vi "Main.vi"(11 "Module Admin":refnum<class "Delacor_lib_QMH_Module Admin.lvclass">) -> ()   [LabVIEW 2016, in "Impedance Data Acquisition and Decoding.lvlib"]
doc: "This template is based off of the Queued Message Handler design pattern and the Queued Message Handler project template that ships with LabVIEW.\n\nThe main difference is that the queue is private to this module and communication between modules is performed via Broadcast and Request events.\n\nRequest events are wrapped in public API methods and are handled in the Event Handling Loop (EHL) of this VI. Any module can register for Broadcast events sent by this module. The EHL generates messages based on user interface actions.\n\nThe Message Handling Loop (MHL) processes messages generated by the EHL, or by other messages. The messages are string values, so new messages can be added easily to the Message Cases case structure in the MHL. Each message cluster can also provide an optional value for Message Data, which is a variant that can be converted to whatever message-specific data is required.\n_____\nBased on Delacor QMH Project Template 5.0.0.82."
uses:
  Impedance Data Acquisition and Decoding.lvlib
  Module Data--cluster.ctl
  <vilib>/Delacor/Delacor QMH/Libraries/Message Queue_class/Delacor_lib_QMH_Message Queue.lvclass
  <vilib>/Delacor/Delacor QMH/Libraries/Message Queue_class/Delacor_lib_QMH_Enqueue Message (Single).vi
  <vilib>/ErrorRing/Error Ring.xnode
  <vilib>/Utility/error.llb/Error Cluster From Error Code.vi
  <vilib>/Delacor/Delacor QMH/Libraries/Module Admin_class/Delacor_lib_QMH_Module Admin.lvclass
  Stop Argument--cluster.ctl
  <vilib>/Utility/miscctls.llb/LVPointTypeDef.ctl
  Stop Acquiring Argument--cluster.ctl
  BusA/FINS3-E BusA Data Acquisition and Decoding/BusA Hardware Configuration.ctl
  FINS-3E Settings Editor/Settings--cluster.ctl
  FINS-3E Settings Editor/Update Application Settings (Reply Payload)--cluster.ctl
  BusB Typedef.ctl
  BusB Hardware Configuration.ctl
  Start Acquiring (Reply Payload)--cluster.ctl
  Start Acquiring Argument--cluster.ctl
  BusD/FINS3-E BusD Data Acquisition and Decoding/BusD Hardware Configuration.ctl
  FINS-3E Settings Editor/Logging Configuration.ctl
  BusB Initialization Parameters.ctl
  BusA/FINS3-E BusA Data Acquisition and Decoding/FCC Parameters.ctl
  IMU/FINS3-E IMU Data Acquisition and Decoding/FINS3-E IMU Hardware Configuration.ctl
  Configurator/FINS3-E Config Hardware Configuration.ctl
  AC 1553/FINS3-E AC Data Acquisition and Decoding/Aircraft Bus Hardware Configuration.ctl
  TERCOM/FINS3-E TERCOM Data Acquisition and Decoding/TERCOM Hardware Configuration.ctl
  DSMAC/FINS3-E DSMAC Data Acquisition and Decoding/DSMAC Hardware Configuration.ctl
  FINS3-E TEL Bus/GPS Hardware Configuration.ctl
  Initialize FINS for FTR Argument--cluster.ctl
  Initialize FINS for Qualification Argument--cluster.ctl
  Settings Editor/Settings Editor.lvlib
  Acquisition/Reg_Map.ctl
  Acquisition/Acquisition.lvlib
  Acquisition/WiBCI16T_Status.ctl
  Acquisition/WiBCI16T_Data.ctl
panel:
  out "error out":errorcluster
  out "Status":string
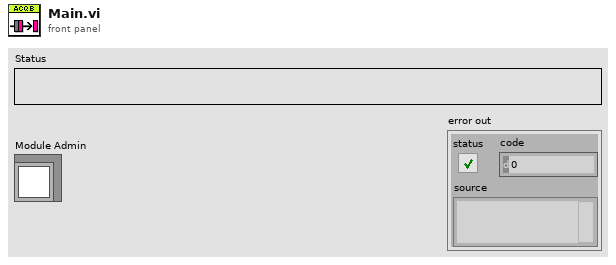
[diagram p1: front panel]
types:
  T1 = typedef "Impedance Data Acquisition and Decoding.lvlib/Request Events--cluster.ctl" = cluster{"Stop Module":refnum<user-event>, "Show Panel":refnum<user-event>, "Hide Panel":refnum<user-event>, "Get Module Execution Status":refnum<user-event>, "Show Diagram":refnum<user-event>, "Stop Acquiring":refnum<user-event>, "Change Settings":refnum<user-event>, "Start Acquiring":refnum<user-event>, "WakeUp Helper Loop":refnum<user-event>, "Initialize FINS":refnum<user-event>, "Initialize FINS for FTR":refnum<user-event>, "Initialize FINS for Qualification":refnum<user-event>}
  T2 = typedef "Settings Editor.lvlib/Broadcast Events--cluster.ctl" = cluster{"Module Did Init":refnum<user-event>, "Status Updated":refnum<user-event>, "Error Reported":refnum<user-event>, "Module Did Stop":refnum<user-event>, "Update Module Execution Status":refnum<user-event>, "Application Settings Updated":refnum<user-event>}
  T3 = typedef "Impedance Data Acquisition and Decoding.lvlib/Broadcast Events--cluster.ctl" = cluster{"Module Did Init":refnum<user-event>, "Status Updated":refnum<user-event>, "Error Reported":refnum<user-event>, "Module Did Stop":refnum<user-event>, "Update Module Execution Status":refnum<user-event>, "Acquisition Stopped":refnum<user-event>, "BusB Raw Data":refnum<user-event>, "BusB Decoded Data Updated":refnum<user-event>, "Acquisition Started":refnum<user-event>, "Read Timeout Error Generation":refnum<user-event>}
  T4 = typedef "Impedance Data Acquisition and Decoding.lvlib/BusB Typedef.ctl" = cluster{"Pitch Rate":dbl, "Roll Rate":dbl, "Roll Angle":dbl, "Yaw Rate":dbl, "True Heading":dbl, "Pitch Angle":dbl, "Y Accel":dbl, "X Accel":dbl, "Z Accel":dbl, "X Gyro Temperature":dbl, "Longitude GPS":dbl, "Latitude GPS":dbl, "Altitude GPS":dbl, "Track Heading GPS":dbl, "Longitude Int":dbl, "Latitude Int":dbl, "Altitude Int":dbl, "FINS System Time":dbl, "East Velocity Int":dbl, "North Velocity Int":dbl, "INS Code Version":dbl, "ModeWord":cluster{"FINS Alg mode":bool, "GPS Data available":bool, "1553 Data available":bool, "Transfer Alignment Successful":bool, "TERCOM Self check OK":bool, "Free Inertial Nav Mode":bool, "TERCOM Data available":bool, "Self Test Request to DSMAC and TERCOM":bool, "ARM Data Available/DSMAC Self-Test OK":bool, "DSMAC valid flag OK":bool, "DSMAC data available":bool, "TERCOM valid flag OK":bool, "GPS aided":bool, "1553 aided":bool, "DSMAC aided":bool, "TERCOM aided":bool, "Aided Nav Mode":bool, " FINS Stdby mode":bool}, "Down Velocity Int":dbl, "Track Heading":dbl, "Y Gyro Temperature":dbl, "Z Gyro Temperature":dbl}
  T5 = enum32{"invalid lock state", "Not Locked", "Locked (No Password)", "Password-protected"}
  T6 = typedef "Impedance Data Acquisition and Decoding.lvlib/Stop Argument--cluster.ctl" = cluster{"Origin":string, "Exit via Stop Module Req?":bool, "Wait for Module to stop?":bool}
  T7 = typedef "Impedance Data Acquisition and Decoding.lvlib/Stop Acquiring Argument--cluster.ctl" = cluster{"Boolean":bool}
  T8 = typedef "FINS-3E Settings Editor.lvlib/Update Application Settings (Reply Payload)--cluster.ctl" = cluster{"Settings":T9, "Update Settings_error":errorcluster}
  T9 = typedef "FINS-3E Settings Editor.lvlib/Settings--cluster.ctl" = cluster{"Logging Configuration":T10, "BusA Hardware Configuration":T11, "BusB Hardware Configuration":T13, "BusD Hardware Configuration":T15, "FINS3-E IMU Hardware Configuration":T16, "FINS3-E Config Hardware Configuration":T17, "DSMAC Hardware Configuration":T18, "TERCOM Hardware Configuration":T19, "A/C Bus Hardware Configuration":T20, "GPS Hardware Configuration":T21, "Equipment Resources":cluster{"Fluke DMM 8846A\nSerial Port":refnum<visa-resource-name>, "CPX400 Serial Port":refnum<k15>, "Temp. Chamber":refnum<visa-resource-name>}}
  T10 = typedef "FINS-3E Settings Editor.lvlib/Logging Configuration.ctl" = cluster{"Log File Base Path":path, "TDMS File Reference":refnum<k34>, "Log File Full Path":path, "Test Rport Full Path":path, "Operator Settings":cluster{"Test Operator":string, "Test Time":timestamp, "Test Location":string, "Unit Under Test":string, "Test Name":string}, "Functionality Test Report Template Path":path, "BusD Logging":enum16{"Limited", "Full"}}
  T11 = typedef "FINS3-E BusA Data Acquisition and Decoding.lvlib/BusA Hardware Configuration.ctl" = cluster{"BusA Serial Port":refnum<visa-resource-name>, "BusA Baud Rate":string, "BusA Bus Update Rate (Hz)":string, "FCC Parameters":T12}
  T12 = typedef "FINS3-E BusA Data Acquisition and Decoding.lvlib/FCC Parameters.ctl" = cluster{"ADU Altitude":dbl, "RA Altitude":dbl}
  T13 = typedef "Impedance Data Acquisition and Decoding.lvlib/BusB Hardware Configuration.ctl" = cluster{"BusB Serial Port":refnum<visa-resource-name>, "BusB Baud Rate":string, "BusB Initialization Parameters":T14}
  T14 = typedef "Impedance Data Acquisition and Decoding.lvlib/BusB Initialization Parameters.ctl" = cluster{"FCC Alignment Pkt":cluster{"Latitude":dbl, "Longitude":dbl, "Altitude":dbl, "Start Alignment":bool, "Alignment Time":u8, "Start Navigation":bool, "Init Alg Parameters":bool}}
  T15 = typedef "FINS3-E BusD Data Acquisition and Decoding.lvlib/BusD Hardware Configuration.ctl" = cluster{"FINS3-E BusD Serial Port":refnum<visa-resource-name>, "FINS3-E BusD Baud Rate":string, "FINS3-E BusD Bus Update Rate (Hz)":string}
  T16 = typedef "FINS3-E IMU Data Acquisition and Decoding.lvlib/FINS3-E IMU Hardware Configuration.ctl" = cluster{"FINS3-E IMU Serial Port":refnum<visa-resource-name>, "FINS3-E IMU Baud Rate":string, "FINS3-E IMU Bus Update Rate (Hz)":string}
  T17 = typedef "FINS3-E Configurator.lvlib/FINS3-E Config Hardware Configuration.ctl" = cluster{"FINS3-E Config Serial Port":refnum<visa-resource-name>, "FINS3-E Config Baud Rate":string}
  T18 = typedef "FINS3-E DSMAC Data Acquisition and Decoding.lvlib/DSMAC Hardware Configuration.ctl" = cluster{"DSMAC Serial Port":refnum<visa-resource-name>, "DSMAC Baud Rate":string, "DSMAC Bus Update Rate (Hz)":string}
  T19 = typedef "FINS3-E TERCOM Data Acquisition and Decoding.lvlib/TERCOM Hardware Configuration.ctl" = cluster{"TERCOM Serial Port":refnum<visa-resource-name>, "TERCOM Baud Rate":string, "TERCOM Bus Update Rate (Hz)":string}
  T20 = typedef "FINS3-E AC Data Acquisition and Decoding.lvlib/Aircraft Bus Hardware Configuration.ctl" = cluster{"A/C Bus Serial Port":refnum<visa-resource-name>, "A/C Bus Baud Rate":string, "A/C Bus Bus Update Rate (Hz)":string, "Aircraft Type":enum16{"Mirage", "JF-17"}}
  T21 = typedef "FINS3-E TEL Bus.lvlib/GPS Hardware Configuration.ctl" = cluster{"GPS Serial Port":refnum<visa-resource-name>, "GPS Baud Rate":string}
  T22 = typedef "Impedance Data Acquisition and Decoding.lvlib/Start Acquiring Argument--cluster.ctl" = cluster{"Wait Notifier":refnum<notifier>, "wait for reply":bool}
  T23 = typedef "Impedance Data Acquisition and Decoding.lvlib/Initialize FINS for FTR Argument--cluster.ctl" = cluster{"Boolean":bool}
  T24 = typedef "Impedance Data Acquisition and Decoding.lvlib/Initialize FINS for Qualification Argument--cluster.ctl" = cluster{"Boolean":bool}
  T25 = typedef "LVPointTypeDef.ctl" = cluster{"Horizontal":i16, "Vertical":i16}
  T26 = enum32{"Invalid", "Standard", "Closed", "Hidden", "Minimized", "Maximized"}
  T27 = typedef "Impedance Data Acquisition and Decoding.lvlib/Start Acquiring (Reply Payload)--cluster.ctl" = cluster{"Start Acquiring_error":errorcluster, "BusB VISA Resource":refnum<visa-resource-name>}
  T28 = typedef "Impedance Data Acquisition and Decoding.lvlib/Module Data--cluster.ctl" = cluster{"WiBCI16T Data":T29}
  T29 = typedef "Acquisition.lvlib/WiBCI16T_Data.ctl" = cluster{"EEG Ch 1":dbl, "EEG Ch 2":dbl, "EEG Ch 3":dbl, "EEG Ch 4":dbl, "EEG Ch 5":dbl, "EEG Ch 6":dbl, "EEG Ch 7":dbl, "EEG Ch 8":dbl, "EEG Ch 9":dbl, "EEG Ch 10":dbl, "EEG Ch 11":dbl, "EEG Ch 12":dbl, "EEG Ch 13":dbl, "EEG Ch 14":dbl, "EEG Ch 15":dbl, "EEG Ch 16":dbl, "X-Accel":i16, "Y-Accel":i16, "Z-Accel":i16, "X-Gyro":i16, "Y-Gyro":i16, "Z-Gyro":i16, "Timer":u32, "Packet ID":u32, "HW Trig1":u8, "SW Trig1":i8, "HW Trig2":u8, "SW Trig2":i8, "WiBCI Status":T30, "Reg Map":T31}
  T30 = typedef "Acquisition.lvlib/WiBCI16T_Status.ctl" = cluster{"Mode Byte":u8, "Ch Config":u8, "Ch Ref Map":u16, "Ch Enable Map":u16, "Temperature":sgl, "Battery":u8, "Version":string}
  T31 = typedef "Acquisition.lvlib/Reg_Map.ctl" = cluster{"ADS1":u8[], "ADS2":u8[]}
  T32 = typedef "FINS3-E BusB Data Acquisition and Decoding.lvlib/BusB Hardware Configuration.ctl" = cluster{"BusB Serial Port":refnum<visa-resource-name>, "BusB Baud Rate":string, "BusB Initialization Parameters":T33}
  T33 = typedef "FINS3-E BusB Data Acquisition and Decoding.lvlib/BusB Initialization Parameters.ctl" = cluster{"FCC Alignment Pkt":cluster{"Latitude":dbl, "Longitude":dbl, "Altitude":dbl, "Start Alignment":bool, "Alignment Time":u8, "Start Navigation":bool, "Init Alg Parameters":bool}}
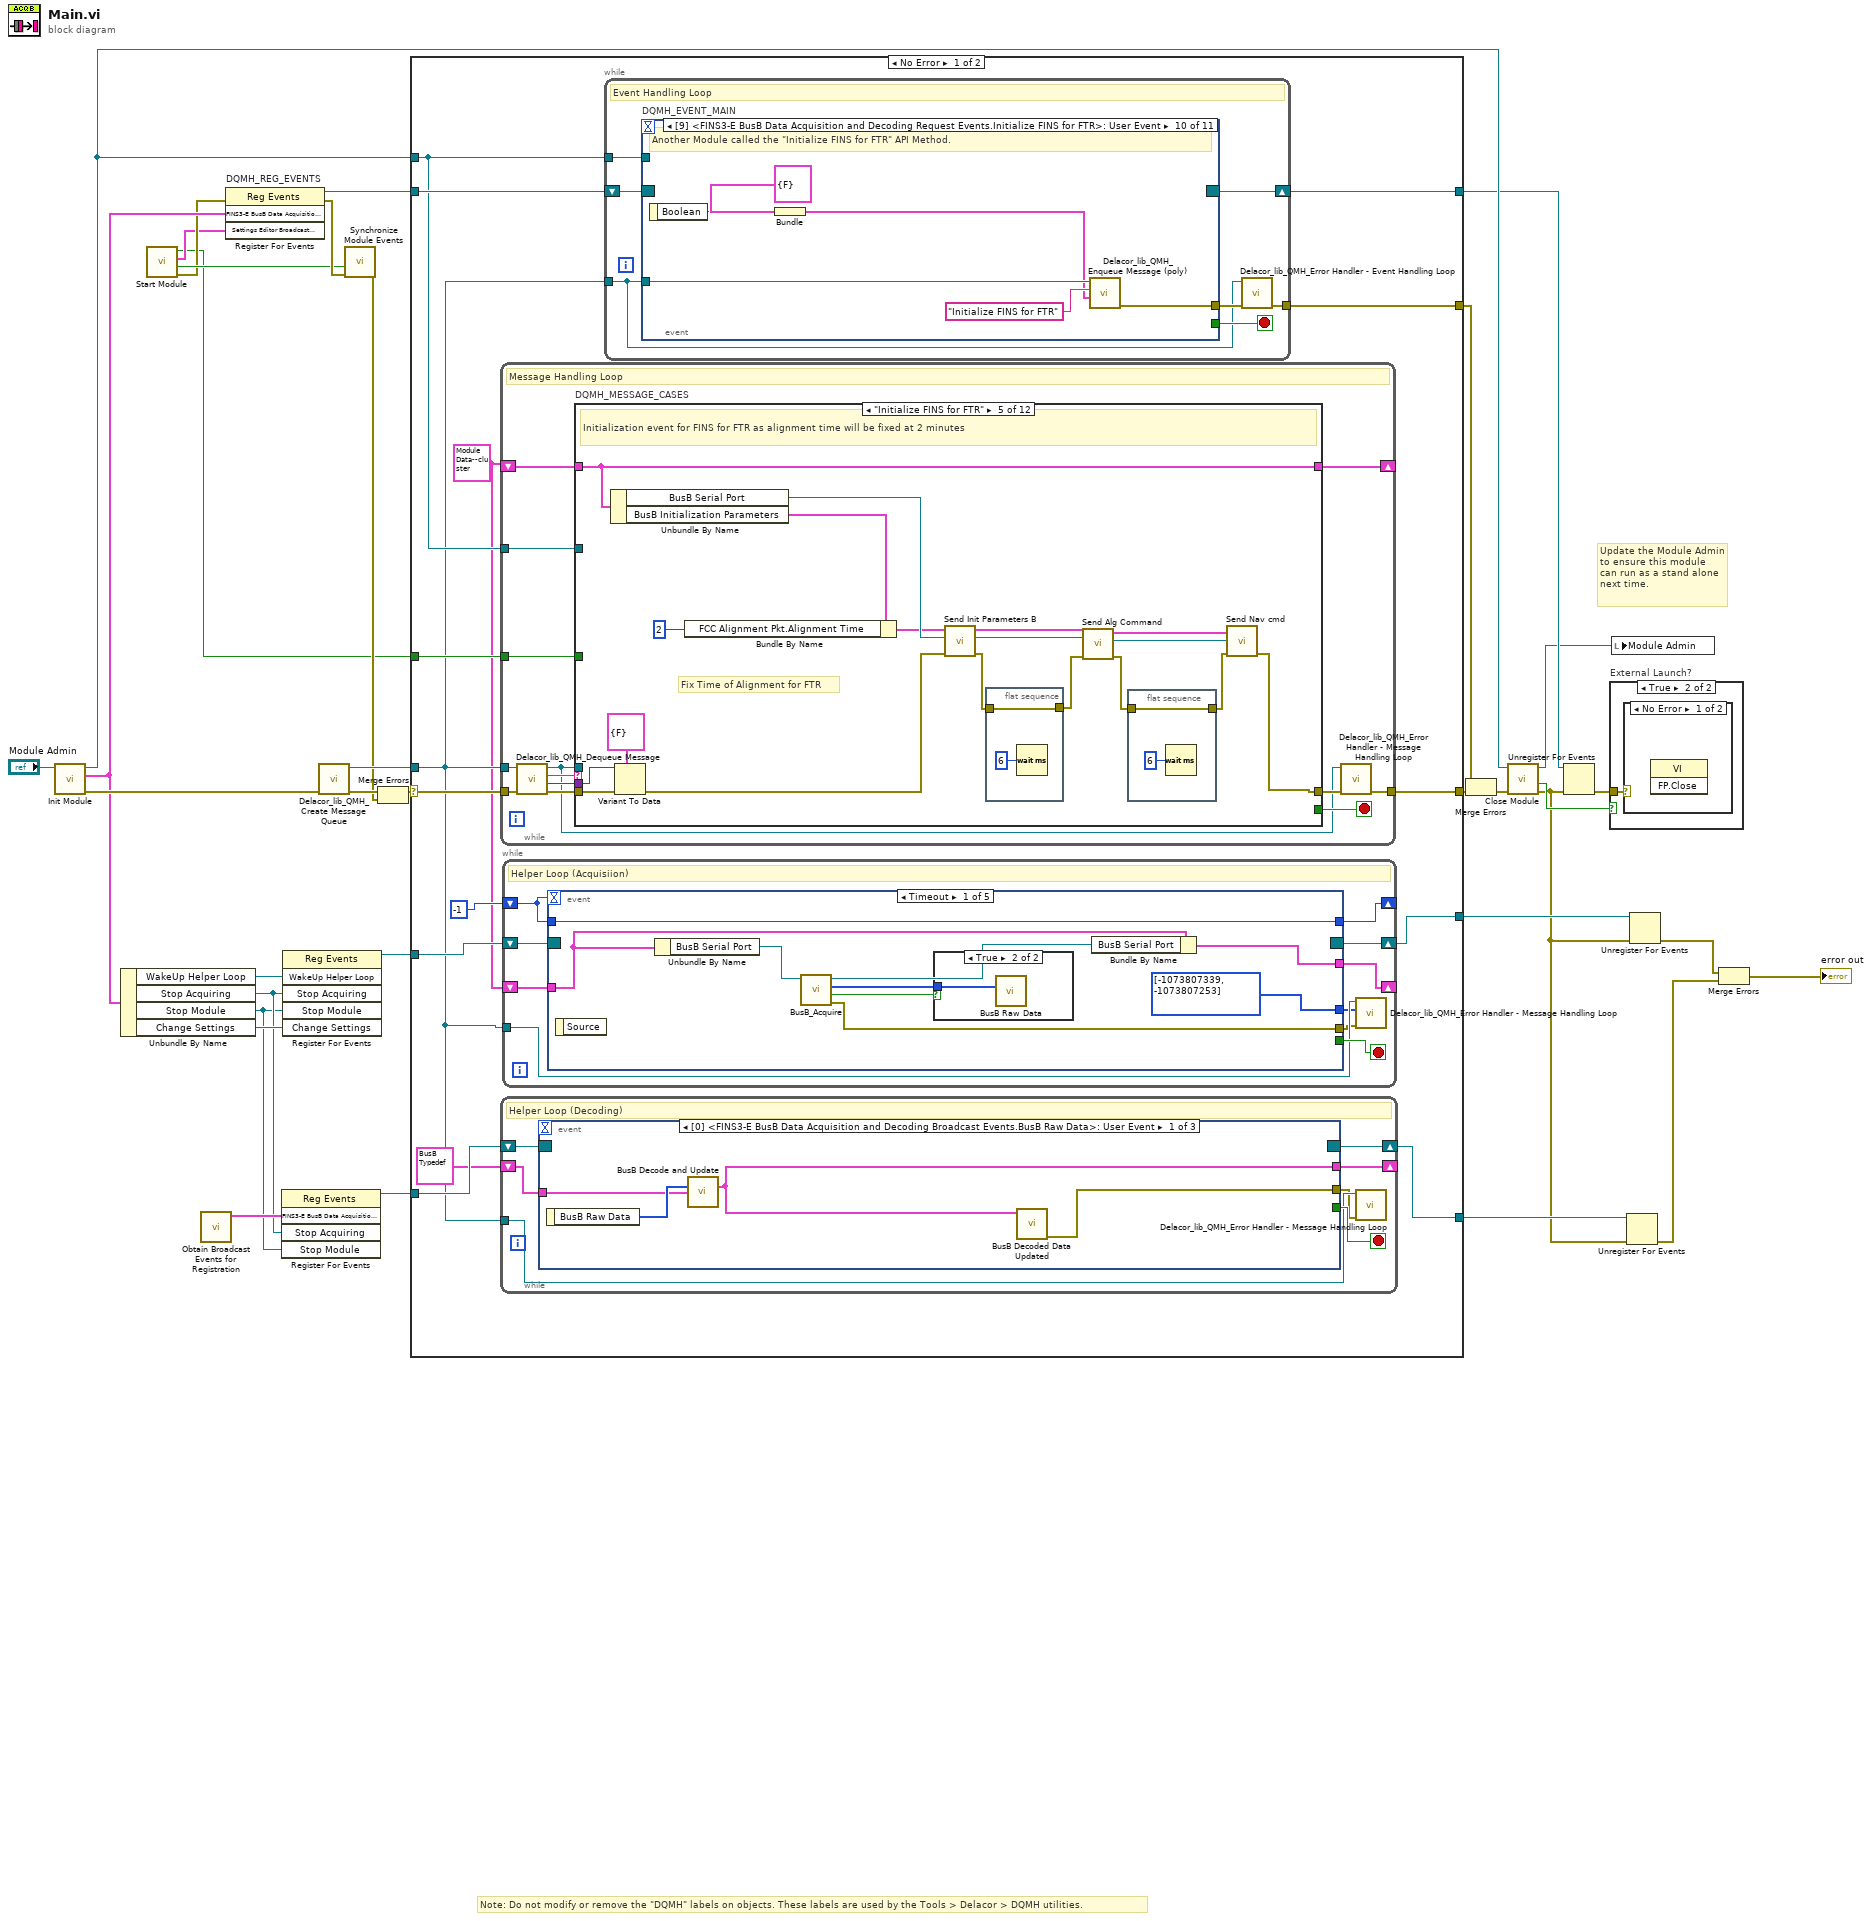
[diagram p0: block diagram]
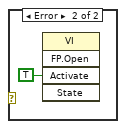
[diagram p3: hidden frame]
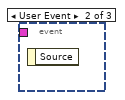
[diagram p4: hidden frame]
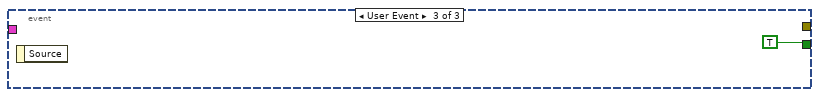
[diagram p5: hidden frame]
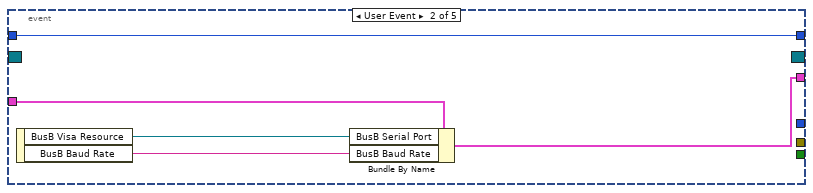
[diagram p7: hidden frame]
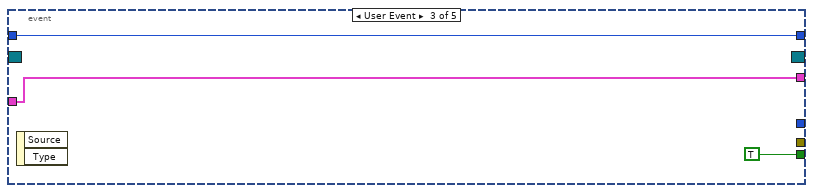
[diagram p8: hidden frame]
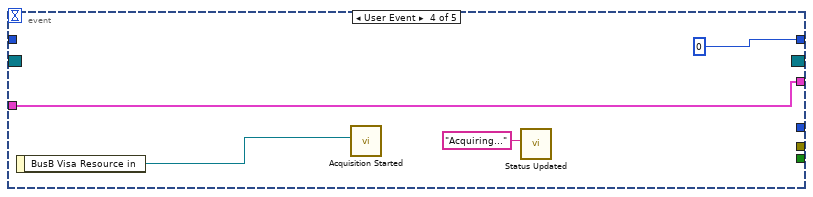
[diagram p9: hidden frame]
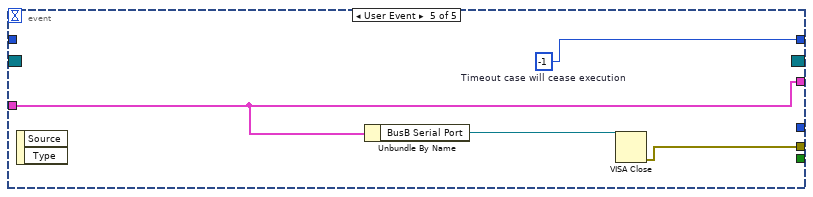
[diagram p10: hidden frame]
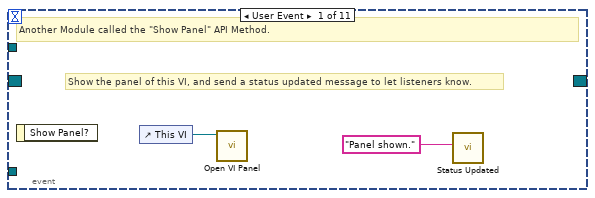
[diagram p11: hidden frame]
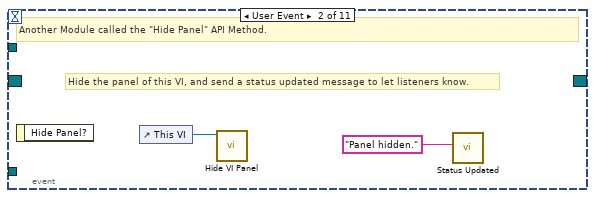
[diagram p12: hidden frame]
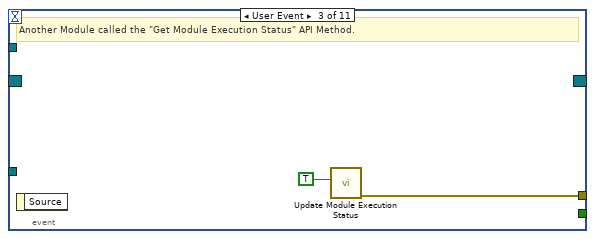
[diagram p13: hidden frame]
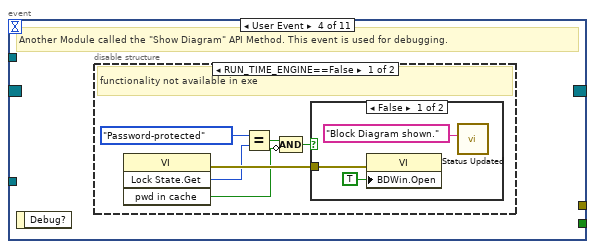
[diagram p14: hidden frame]
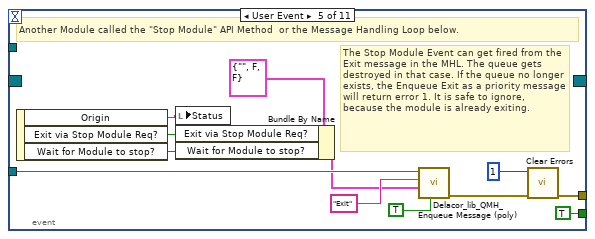
[diagram p17: hidden frame]
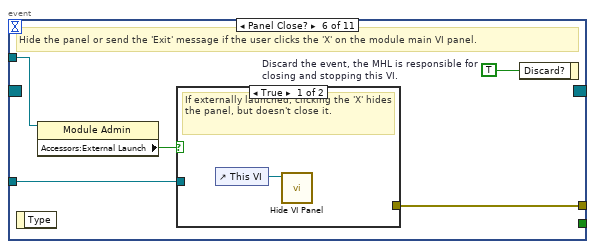
[diagram p18: hidden frame]
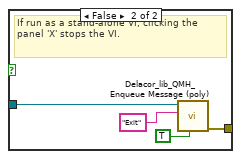
[diagram p19: hidden frame]
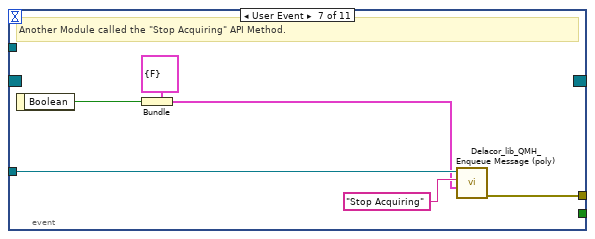
[diagram p20: hidden frame]
diagram:
  # "Note: Do not modify or remove the \"DQMH\" labels on objects. These labels are used by the Tools > Delacor > DQMH utilities."
  # "Update the Module Admin to ensure this module can run as a stand alone next time."
  n1 = call "Init Module.vi"("Singleton Module Admin in"="Module Admin") -> ("error out"=w33:errorcluster, "FINS3-E BusB Data Acquisition and Decoding Request Events"=w20:T1, "Singleton Module Admin out"=w27:refnum<class "Delacor_lib_QMH_Module Admin.lvclass">)  [unwired: 8 in]
  n2 = Unbundle By Name(w20) -> ("WakeUp Helper Loop"=w19:refnum<user-event>, "Stop Acquiring"=w15:refnum<user-event>, "Stop Module"=w14:refnum<user-event>, "Change Settings"=w18:refnum<user-event>)
  n3 = call "Start Module.vi"() -> ("error out"=w3:errorcluster, "Wait for Event Sync?"=w4:bool, "Settings Editor Broadcast Events"=w2:T2, "Module Was Already Running?"=w1:bool)  [unwired: 8 in]
  n4 = call "Obtain Broadcast Events for Registration.vi"() -> ("FINS3-E BusB Data Acquisition and Decoding Broadcast Events"=w16:T3)  [unwired: 9 in, 2 out]
  n5 = register-events "DQMH_REG_EVENTS"(error in=w3, w20, w2) -> (reference out=w25:refnum<event-registration>, error out=w6:errorcluster)  [unwired: 1 in]
  n6 = register-events(w16, w15, w14) -> (reference out=w13:refnum<event-registration>)  [unwired: 2 in, 1 out]
  n7 = register-events(w19, w15, w14, w18) -> (reference out=w17:refnum<event-registration>)  [unwired: 2 in, 1 out]
  n8 = call <vilib>:"Delacor_lib_QMH_Create Message Queue.vi"("error in"=w33) -> ("error out"=w29:errorcluster, "Message Queue"=w24:refnum<class "Delacor_lib_QMH_Message Queue.lvclass">)  [unwired: 9 in]
  n9 = call "Synchronize Module Events.vi"("error in (no error)"=w6, "Wait for Event Sync?"=w4) -> ("error out"=w5:errorcluster)  [unwired: 9 in]
  n10 = Merge Errors(w29, w5) -> (w28:errorcluster)
  n11 = case shown="No Error" w28 {
    selector: w28 -> [w47 w358]
    tunnel: [w49 w357] -> w34
    tunnel: [w46 w363] -> w26
    tunnel: w25 -> [w45 w363]
    tunnel: w24 -> [w37 w356]
    tunnel: [w48 _] -> w32
    tunnel: w27 -> [w44 w359]
    tunnel: w1 -> [w43 _]
    tunnel: w17 -> [w42 w355]
    tunnel: w13 -> [w40 w354]
    tunnel: [w39 w355] -> w12
    tunnel: [w38 w354] -> w11
    frame No Error {
      w35 = T28 {"WiBCI16T Data"={"EEG Ch 1"=0.0, "EEG Ch 2"=0.0, "EEG Ch 3"=0.0, "EEG Ch 4"=0.0, "EEG Ch 5"=0.0, "EEG Ch 6"=0.0, "EEG Ch 7"=0.0, "EEG Ch 8"=0.0, "EEG Ch 9"=0.0, "EEG Ch 10"=0.0, "EEG Ch 11"=0.0, "EEG Ch 12"=0.0, "EEG Ch 13"=0.0, "EEG Ch 14"=0.0, "EEG Ch 15"=0.0, "EEG Ch 16"=0.0, "X-Accel"=0, "Y-Accel"=0, "Z-Accel"=0, "X-Gyro"=0, "Y-Gyro"=0, "Z-Gyro"=0, "Timer"=0, "Packet ID"=0, "HW Trig1"=0, "SW Trig1"=0, "HW Trig2"=0, "SW Trig2"=0, "WiBCI Status"={"Mode Byte"=0, "Ch Config"=0, "Ch Ref Map"=0, "Ch Enable Map"=0, "Temperature"=0.0, "Battery"=0, "Version"="460800"}, "Reg Map"={"ADS1"=[], "ADS2"=[]}}} ("Data Cluster")
      n12 = while {
        tunnel: w37 -> [w177]
        shift-right: [w181] -> _
        shift-left: w35 -> [w182]
        tunnel: w47 -> [w185]
        tunnel: [w183] -> w49
        tunnel: w44 -> [w175]
        tunnel: w43 -> [w174]
        stop <- w180 stop-if-true
        # "Message Handling Loop"
        n13 = call-dynamic "Delacor_lib_QMH_Dequeue Message.vi"("error in"=w185, "Message Queue in"=w177) -> ("error out"=w184:errorcluster, "Message Data"=w178:variant, "Message"=w179:string, "Message Queue out"=w176:refnum<class "Delacor_lib_QMH_Message Queue.lvclass">)  [unwired: 6 in]
        n14 = case "DQMH_MESSAGE_CASES" shown="\"Initialize FINS for FTR\"" w179 {
          selector: w179 -> [_ _ _ _ _ _ _ _ _ _ _ w341]
          tunnel: w176 -> [_ _ _ _ _ _ _ _ _ w305 w334 _]
          tunnel: w184 -> [w206 w210 w224 w240 w258 w280 w287 w299 w301 w312 w337 w343]
          tunnel: [w204 w210 w214 w237 w247 w266 w286 w294 w301 w308 w336 w344] -> w186
          tunnel: w182 -> [w195 w209 w217 w233 w246 w265 w285 w289 w300 w307 w321 w342]
          tunnel: [w194 w209 w216 w233 w246 w265 w285 w288 w300 w307 w321 w342] -> w181
          tunnel: [_ _ _ _ _ _ _ _ _ _ w333 _] -> w180
          tunnel: w178 -> [_ _ w223 w239 w257 w279 _ w297 _ w306 w332 _]
          tunnel: w175 -> [w196 _ _ _ _ _ _ _ _ w304 w327 _]
          tunnel: w174 -> [_ _ _ _ _ _ _ _ _ _ w325 _]
          frame "Initialize" {
            (unwired) "Initial Message" ("Initial Message")
            # "Initialize - Any operation that needs to be done before the module can receive messages. Synchronize Caller Events.vi will inform Start Module.vi that the module has launched and is ready to receive messages. Module Did Init.vi will broadcast that the module initialized."
            n15 = call "Synchronize Caller Events.vi"("error in (no error)"=w206, "Singleton Module Admin in"=w196) -> ("error out"=w205:errorcluster, "Singleton Module Admin out"=w191:refnum<class "Delacor_lib_QMH_Module Admin.lvclass">)  [unwired: 8 in]
            n16 = call "Update Application Settings.vi"("wait for reply (T)"=TRUE) -> ("Reply Payload"=w189:T8)  [unwired: 8 in, 2 out]
            n17 = property class="Module Admin"(reference=w191) -> ("Accessors:External Launch"=w200:bool)  [unwired: 1 in, 2 out]
            n18 = Unbundle By Name(w189) -> ("Settings.BusB Hardware Configuration"=w188:T32)
            n19 = Select(t=T26."Hidden" ("State"), s=w200, f=T26."Standard" ("State")) -> (s? t:f=w197:T26)
            n20 = call "Module Name--constant.vi"() -> ("Module Name"=w203:string)  [unwired: 11 in]
            n21 = property class="VI"("Front Panel.Title"=w203) -> (reference out=w202:refnum<vi>, error out=w208:errorcluster)  [unwired: 2 in]
            n22 = Bundle By Name(cluster=w195, "BusB Hardware Configuration"=w188) -> (w194:T28)
            n23 = call "Module Name--constant.vi"() -> ("Module Name"=w192:string)  [unwired: 11 in]
            n24 = invoke class="VI" method="FP.Open"(reference=w202, error in=w208, "State"=w197) -> (reference out=w201:refnum<vi>, error out=w207:errorcluster)  [unwired: 2 in, 3 out]
            n25 = call "Module Did Init.vi"("error in (no error)"=w205, "Initialized?"=TRUE, "Origin"=w192) -> ("error out"=w204:errorcluster)  [unwired: 8 in]
            n26 = invoke class="VI" method="FP.Center"(reference=w201, error in=w207) -> ()  [unwired: 1 in, 3 out]
            n27 = property on="Pane" class="Pane"("Origin"=T25 {"Horizontal"=0, "Vertical"=0}) -> ()  [unwired: 2 in, 2 out]
          }
          frame "--- Module Specific ---" {
            # "Separator -- The following cases handle messages specific to this Module."
          }
          frame "Start Acquiring" {
            n28 = Variant To Data(error in=w224, type=T22 {"Wait Notifier"=refnum, "wait for reply"=FALSE} ("Start Acquiring Argument"), Variant=w223) -> (data=w221:T22, error out=w215:errorcluster)
            n29 = in-place {
              in-place-border: w215 -> [w231]
              in-place-border: [w226] -> w213
              in-place-border: [w225] -> w212
              n30 = in-place-cluster #1(w217) -> ("BusB Serial Port"=w229:refnum<visa-resource-name>, "BusB Baud Rate"=w228:string)
              n31 = call "BusB_Initialize Hardware References.vi"("error in (no error)"=w231, "BusB Baud Rate"=w228, "BusB Visa Resource in"=w229) -> ("error out"=w230:errorcluster, "BusB Visa Resource out"=w227:refnum<visa-resource-name>)  [unwired: 6 in, 1 out]
              n32 = call "BusB_Configure Hardware.vi"("error in (no error)"=w230, "BusB Visa Resource in"=w227) -> ("error out"=w225:errorcluster, "BusB Visa Resource out"=w226:refnum<visa-resource-name>)  [unwired: 8 in]
              n33 = in-place-cluster #1("BusB Serial Port"=w226, "BusB Baud Rate"=w228) -> (w216:T28)
            }
            n34 = call "Read Timeout Error Generation.vi"("error in (no error)"=w212) -> ("error out"=w211:errorcluster)  [unwired: 10 in]
            n35 = Unbundle By Name(w221) -> ("Wait Notifier"=w220:refnum<notifier>)
            n36 = Bundle By Name(cluster=T27 {"Start Acquiring_error"={"status"=FALSE, "code"=0, "source"=""}, "BusB VISA Resource"=""} ("Start Acquiring (Reply Payload)"), "BusB VISA Resource"=w213, "Start Acquiring_error"=w211) -> (w219:T27)
            n37 = call "WakeUp Helper Loop.vi"("error in (no error)"=w211, "BusB Visa Resource in"=w213) -> ("error out"=w214:errorcluster)  [unwired: 9 in]
            n38 = Send Notification(notification=w219, notifier=w220) -> ()  [unwired: 1 in, 2 out]
          }
          frame "Stop Acquiring" {
            n39 = Variant To Data(error in=w240, type=T7 {"Boolean"=FALSE} ("Stop Acquiring Argument"), Variant=w239) -> (error out=w234:errorcluster)  [unwired: 1 out]
            n40 = Unbundle By Name(w233) -> ("BusB Serial Port"=w232:refnum<visa-resource-name>)
            n41 = call "BusB_Stop Acquisition.vi"("error in (no error)"=w234, "BusB Visa Resource"=w232) -> ("error out"=w236:errorcluster)  [unwired: 9 in]
            n42 = call "Status Updated.vi"("error in (no error)"=w234, "Status"="Acquisition Stopped") -> ()  [unwired: 9 in, 1 out]
            n43 = call "Acquisition Stopped.vi"("error in (no error)"=w236) -> ("error out"=w237:errorcluster)  [unwired: 10 in]
          }
          frame "Initialize FINS for FTR" {
            # "Fix Time of Alignment for FTR"
            # "Initialization event for FINS for FTR as alignment time will be fixed at 2 minutes"
            n44 = Unbundle By Name(w246) -> ("BusB Serial Port"=w245:refnum<visa-resource-name>, "BusB Initialization Parameters"=w243:T14)
            n45 = Variant To Data(error in=w258, type=T23 {"Boolean"=FALSE} ("Initialize FINS for FTR Argument"), Variant=w257) -> (error out=w244:errorcluster)  [unwired: 1 out]
            n46 = Bundle By Name(cluster=w243, "FCC Alignment Pkt.Alignment Time"=u8 2) -> (w241:T14)
            n47 = call "Send Init Parameters B.vi"("error in"=w244, "BusB Serial Port"=w245, "BusB Hardware Configuration.BusB Initialization Parameters"=w241) -> ("error out"=w255:errorcluster, "BusB Serial Port out"=w254:refnum<visa-resource-name>, "BusB Hardware Configuration.BusB Initialization Parameters 2"=w249:T14)  [unwired: 6 in]
            n48 = flat-sequence {
              tunnel: w255 -> [w261]
              tunnel: [w261] -> w253
              frame #0 {
                n49 = Wait (ms)(milliseconds to wait=u32 6) -> ()  [unwired: 1 out]
              }
            }
            n50 = call "Send Alg Command.vi"("error in"=w253, "BusB Serial Port"=w254, "BusB Hardware Configuration.BusB Initialization Parameters"=w249) -> ("error out"=w252:errorcluster, "BusB Serial Port out"=w251:refnum<visa-resource-name>, "BusB Hardware Configuration.BusB Initialization Parameters 2"=w248:T14)  [unwired: 6 in]
            n51 = flat-sequence {
              tunnel: w252 -> [w259]
              tunnel: [w259] -> w250
              frame #0 {
                n52 = Wait (ms)(milliseconds to wait=u32 6) -> ()  [unwired: 1 out]
              }
            }
            n53 = call "Send Nav cmd.vi"("error in"=w250, "BusB Serial Port"=w251, "BusB Hardware Configuration.BusB Initialization Parameters"=w248) -> ("error out"=w247:errorcluster)  [unwired: 6 in, 2 out]
          }
          frame "Initialize FINS for Qualification" {
            # "Fix Time of Alignment for Qualification"
            # "FINS is initialized with alignment time of 10 minutes even if Settings are otherwise"
            n54 = Variant To Data(error in=w280, type=T24 {"Boolean"=FALSE} ("Initialize FINS for Qualification Argument"), Variant=w279) -> (error out=w267:errorcluster)  [unwired: 1 out]
            n55 = Unbundle By Name(w265) -> ("BusB Serial Port"=w263:refnum<visa-resource-name>, "BusB Initialization Parameters"=w264:T14)
            n56 = Bundle By Name(cluster=w264, "FCC Alignment Pkt.Alignment Time"=u8 10) -> (w268:T14)
            n57 = call "Send Init Parameters B.vi"("error in"=w267, "BusB Serial Port"=w263, "BusB Hardware Configuration.BusB Initialization Parameters"=w268) -> ("error out"=w277:errorcluster, "BusB Serial Port out"=w276:refnum<visa-resource-name>, "BusB Hardware Configuration.BusB Initialization Parameters 2"=w271:T14)  [unwired: 6 in]
            n58 = flat-sequence {
              tunnel: w277 -> [w283]
              tunnel: [w283] -> w275
              frame #0 {
                n59 = Wait (ms)(milliseconds to wait=u32 6) -> ()  [unwired: 1 out]
              }
            }
            n60 = call "Send Alg Command.vi"("error in"=w275, "BusB Serial Port"=w276, "BusB Hardware Configuration.BusB Initialization Parameters"=w271) -> ("error out"=w274:errorcluster, "BusB Serial Port out"=w273:refnum<visa-resource-name>, "BusB Hardware Configuration.BusB Initialization Parameters 2"=w270:T14)  [unwired: 6 in]
            n61 = flat-sequence {
              tunnel: w274 -> [w281]
              tunnel: [w281] -> w272
              frame #0 {
                n62 = Wait (ms)(milliseconds to wait=u32 6) -> ()  [unwired: 1 out]
              }
            }
            n63 = call "Send Nav cmd.vi"("error in"=w272, "BusB Serial Port"=w273, "BusB Hardware Configuration.BusB Initialization Parameters"=w270) -> ("error out"=w266:errorcluster)  [unwired: 6 in, 2 out]
          }
          frame "---Copy This Frame---" {
            # "Duplicate this frame when creating new messages.  Change this comment in the duplicated frame to describe this message."
            n64 = Merge Errors(w287) -> (w286:errorcluster)
          }
          frame "Update Settings" {
            n65 = Variant To Data(error in=w299, type=T8 {"Settings"={"Logging Configuration"={"Log File Base Path"=path "", "TDMS File Reference"=refnum, "Log File Full Path"=path "", "Test Rport Full Path"=path "", "Operator Settings"={"Test Operator"="", "Test Time"=timestamp(0 s since 1904-01-01), "Test Location"="", "Unit Under Test"="", "Test Name"="Functionality Test"}, "Functionality Test Report Template Path"=path "", "BusD Logging"=enum."Limited"}, "BusA Hardware Configuration"={"BusA Serial Port"="", "BusA Baud Rate"="", "BusA Bus Update Rate (Hz)"="", "FCC Parameters"={"ADU Altitude"=0.0, "RA Altitude"=0.0}}, "BusB Hardware Configuration"={"BusB Serial Port"="", "BusB Baud Rate"="460800", "BusB Initialization Parameters"={"FCC Alignment Pkt"={"Latitude"=0.0, "Longitude"=0.0, "Altitude"=0.0, "Start Alignment"=FALSE, "Alignment Time"=0, "Start Navigation"=FALSE, "Init Alg Parameters"=FALSE}}}, "BusD Hardware Configuration"={"FINS3-E BusD Serial Port"="COM4", "FINS3-E BusD Baud Rate"="460800", "FINS3-E BusD Bus Update Rate (Hz)"=""}, "FINS3-E IMU Hardware Configuration"={"FINS3-E IMU Serial Port"="COM3", "FINS3-E IMU Baud Rate"="460800", "FINS3-E IMU Bus Update Rate (Hz)"=""}, "FINS3-E Config Hardware Configuration"={"FINS3-E Config Serial Port"="COM3", "FINS3-E Config Baud Rate"="460800"}, "DSMAC Hardware Configuration"={"DSMAC Serial Port"="COM3", "DSMAC Baud Rate"="460800", "DSMAC Bus Update Rate (Hz)"=""}, "TERCOM Hardware Configuration"={"TERCOM Serial Port"="COM3", "TERCOM Baud Rate"="460800", "TERCOM Bus Update Rate (Hz)"=""}, "A/C Bus Hardware Configuration"={"A/C Bus Serial Port"="COM3", "A/C Bus Baud Rate"="460800", "A/C Bus Bus Update Rate (Hz)"="", "Aircraft Type"=enum."Mirage"}, "GPS Hardware Configuration"={"GPS Serial Port"="", "GPS Baud Rate"="115200"}, "Equipment Resources"={"Fluke DMM 8846A\nSerial Port"="", "CPX400 Serial Port"="", "Temp. Chamber"=""}}, "Update Settings_error"={"status"=FALSE, "code"=0, "source"=""}} ("Settings Updated Argument"), Variant=w297) -> (data=w291:T8, error out=w298:errorcluster)
            n66 = Unbundle By Name(w291) -> ("Settings.BusB Hardware Configuration"=w290:T13)
            n67 = Unbundle By Name(w291) -> ("Settings.BusB Hardware Configuration.BusB Serial Port"=w295:refnum<visa-resource-name>, "Settings.BusB Hardware Configuration.BusB Baud Rate"=w296:string)
            n68 = Bundle By Name(cluster=w289, "BusB Hardware Configuration"=w290) -> (w288:T28)
            n69 = call "Change Settings.vi"("error in (no error)"=w298, "BusB Bus Update Rate (Hz)"=w296, "BusB Visa Resource"=w295) -> ("error out"=w294:errorcluster)  [unwired: 8 in]
            n70 = call "Status Updated.vi"("error in (no error)"=w294, "Status"="Settings Updated ...") -> ()  [unwired: 9 in, 1 out]
          }
          frame "--- Exit and Error Handling---" {
            # "Separator - The following cases handle errors and exit messages."
          }
          frame "Error" {
            # "#CodeRecommended - If you ever change the name of this \"Error\" message, you'll need to update the name in the Check Loop Error.vi as well."
            # "#CodeRecommended - If the module is running in standalone mode (External Launch = FALSE), this code will pop up an error dialog and call the 'Exit' message if an error occurs. Add more fine-grained error handling here."
            # "Error - Check the error message data and respond accordingly. This message is sent by the \"Error Handler\" VIs at the end of each loop in this application."
            n71 = property class="Module Admin"(reference=w304) -> ("Accessors:External Launch"=w303:bool)  [unwired: 1 in, 2 out]
            n72 = Variant To Data(error in=w312, type=errorcluster {"status"=FALSE, "code"=0, "source"=""} ("error constant"), Variant=w306) -> (data=w313:errorcluster, error out=w310:errorcluster)
            n73 = call "Module Name--constant.vi"() -> ("Module Name"=w302:string)  [unwired: 11 in]
            n74 = call "Error Reported.vi"("Additional Information"=w302, "Error"=w313) -> ()  [unwired: 9 in, 1 out]
            n75 = case shown="False" w303 {
              tunnel: [w318 _] -> w309
              tunnel: w305 -> [w316 _]
              tunnel: w313 -> [w317 _]
              frame False {
                # "If the module is running standalone, then pop up an error dialog and call the \"Exit\" message."
                n76 = call <vilib>:"Simple Error Handler.vi"("error in (no error)"=w317) -> ()  [unwired: 4 in, 5 out]
                n77 = call-poly <vilib>:"Delacor_lib_QMH_Enqueue Message (poly).vi"("Priority Message? (F)"=TRUE, "Message"="Exit", "Message Queue in"=w316) -> ("error out"=w318:errorcluster)  [unwired: 7 in, 1 out]
              }
              frame True {
                # "If the module was launched externally, calling the Error Reported broadcast VI is the only action performed by the \"Error\" message. The module's caller can then process the error appropriately."
              }
            }
            n78 = Merge Errors(w310, w309) -> (w308:errorcluster)
            n79 = local write "error out"(w308) -> ()
          }
          frame "Exit" {
            w331 = 91  # 91: not all Exit messages will have an argument
            w333 = TRUE  # Stop the VI
            # "Release the message queue reference"
            # "Exit - Exit the application."
            n80 = Variant To Data(error in=w337, type=T6 {"Origin"="", "Exit via Stop Module Req?"=FALSE, "Wait for Module to stop?"=FALSE} ("Stop Argument"), Variant=w332) -> (data=w329:T6, error out=w335:errorcluster)
            n81 = call <vilib>:"Clear Errors.vi"("error in (no error)"=w335, "specific error code to clear (0: all)"=w331) -> ("error out"=w324:errorcluster)  [unwired: 4 in, 1 out]
            n82 = Unbundle By Name(w321) -> ("BusB Serial Port"=w320:refnum<visa-resource-name>)
            n83 = call "Module Name--constant.vi"() -> ("Module Name"=w319:string)  [unwired: 11 in]
            n84 = control-ref of="This VI"() -> (w328:refnum<vi>)
            n85 = case shown="False" w325 {
              tunnel: w319 -> [w338 _]
              frame False {
                n86 = call "Stop Module.vi"("Wait for Module to Stop? (F)"=TRUE, "Origin"=w338) -> ()  [unwired: 9 in, 1 out]
              }
              frame True {
                # "Another Module is\nin charge of stopping Settings Editor"
              }
            }
            n87 = call "Handle Exit.vi"("Stop Argument"=w329, "Admin in"=w327, "VI reference"=w328) -> ("error out"=w326:errorcluster)  [unwired: 7 in, 1 out]
            n88 = call "BusB_Close Hardware References.vi"("BusB VISA resource"=w320) -> ("error out"=w322:errorcluster)  [unwired: 9 in, 1 out]
            n89 = call-dynamic "Delacor_lib_QMH_Release Message Queue.vi"("error in"=w324, "Message Queue"=w334) -> ("error out"=w323:errorcluster)  [unwired: 9 in]
            n90 = Merge Errors(w326, w322, w323) -> (w336:errorcluster)
          }
          frame Default {
            # "'Default' case only runs if there is a message that isn't defined in any of the other cases.  Output a programming error."
            n91 = call "Module Name--constant.vi"() -> ("Module Name"=w340:string)  [unwired: 11 in]
            n92 = xnode "Error Ring"("parameter 0"=w341, "parameter 1"=w340) -> ("error out"=w345:errorcluster)
            n93 = Merge Errors(w343, w345) -> (w344:errorcluster)
          }
        }
        n94 = call-dynamic "Delacor_lib_QMH_Error Handler - Message Handling Loop.vi"("error in"=w186, "Message Queue in"=w176) -> ("dup error in"=w183:errorcluster)  [unwired: 8 in, 1 out]
      }
      n95 = while {
        shift-right: [w55] -> w38
        shift-left: w40 -> [w56]
        tunnel: w37 -> [w53]
        shift-right: [w51] -> _
        shift-left: T4 {"Pitch Rate"=0.0, "Roll Rate"=0.0, "Roll Angle"=0.0, "Yaw Rate"=0.0, "True Heading"=0.0, "Pitch Angle"=0.0, "Y Accel"=0.0, "X Accel"=0.0, "Z Accel"=0.0, "X Gyro Temperature"=0.0, "Longitude GPS"=0.0, "Latitude GPS"=0.0, "Altitude GPS"=0.0, "Track Heading GPS"=0.0, "Longitude Int"=0.0, "Latitude Int"=0.0, "Altitude Int"=0.0, "FINS System Time"=0.0, "East Velocity Int"=0.0, "North Velocity Int"=0.0, "INS Code Version"=0.0, "ModeWord"={"FINS Alg mode"=FALSE, "GPS Data available"=FALSE, "1553 Data available"=FALSE, "Transfer Alignment Successful"=FALSE, "TERCOM Self check OK"=FALSE, "Free Inertial Nav Mode"=FALSE, "TERCOM Data available"=FALSE, "Self Test Request to DSMAC and TERCOM"=FALSE, "ARM Data Available/DSMAC Self-Test OK"=FALSE, "DSMAC valid flag OK"=FALSE, "DSMAC data available"=FALSE, "TERCOM valid flag OK"=FALSE, "GPS aided"=FALSE, "1553 aided"=FALSE, "DSMAC aided"=FALSE, "TERCOM aided"=FALSE, "Aided Nav Mode"=FALSE, " FINS Stdby mode"=FALSE}, "Down Velocity Int"=0.0, "Track Heading"=0.0, "Y Gyro Temperature"=0.0, "Z Gyro Temperature"=0.0} ("BusB TypeDef out") -> [w50]
        stop <- w54 stop-if-true
        # "Helper Loop (Decoding)"
        n96 = event shown="[0] <FINS3-E BusB Data Acquisition and Decoding Broadcast Events.BusB Raw Data>: User Event" {
          selector: w56 -> [_ _ _]
          dyn-events: [_ _ _] -> w55
          timeout: _ -> [_ _ _]
          tunnel: [_ _ TRUE] -> w54
          tunnel: [w59 _ _] -> w52
          tunnel: [w57 _ _] -> w51
          tunnel: w50 -> [w58 _ _]
          event User Event {
            n97 = event-data() -> ("BusB Raw Data"=w60:u8[])  [unwired: 1 in]
            n98 = call "BusB Decode and Update.vi"("In"=w60, "BusB TypeDef"=w58) -> ("BusB TypeDef out"=w57:T4)  [unwired: 12 in, 1 out]
            n99 = call "BusB Decoded Data Updated.vi"("BusB TypeDef"=w57) -> ("error out"=w59:errorcluster)  [unwired: 10 in]
          }
          event User Event {
            n100 = event-data() -> ()  [unwired: 1 in, 1 out]
          }
          event User Event {
            n101 = event-data() -> ()  [unwired: 1 in, 1 out]
          }
        }
        n102 = call-dynamic "Delacor_lib_QMH_Error Handler - Message Handling Loop.vi"("error in"=w52, "Message Queue in"=w53) -> ()  [unwired: 8 in, 2 out]
      }
      n103 = while {
        shift-right: [w70] -> w39
        shift-left: w42 -> [w71]
        shift-right: [w68] -> _
        shift-left: -1 -> [w69]
        shift-right: [w66] -> _
        shift-left: w35 -> [w67]
        tunnel: w37 -> [w64]
        stop <- w65 stop-if-true
        # "Helper Loop (Acquisiion)"
        n104 = event shown="[0] Timeout" {
          selector: w71 -> [_ _ _ _ _]
          dyn-events: [_ _ _ _ _] -> w70
          timeout: w69 -> [_ _ _ _ _]
          tunnel: w69 -> [w80 w82 w88 _ _]
          tunnel: [w80 w82 w88 0 w97] -> w68
          tunnel: w67 -> [w78 w84 w87 w92 w96]
          tunnel: [w77 w83 w87 w92 w96] -> w66
          tunnel: [_ _ TRUE _ _] -> w65
          tunnel: [w76 _ _ _ w94] -> w63
          tunnel: [i32[] [-1073807339, -1073807253] _ _ _ _] -> w62
          event Timeout {
            n105 = event-data() -> ()  [unwired: 1 in, 1 out]
            n106 = Unbundle By Name(w78) -> ("BusB Serial Port"=w79:refnum<visa-resource-name>)
            n107 = call "BusB_Acquire.vi"("BusB VISA resource in"=w79) -> ("error out"=w76:errorcluster, "Match & Update"=w74:bool, "BusB Raw Data"=w73:u8[], "BusB VISA resource out"=w75:refnum<visa-resource-name>)  [unwired: 7 in]
            n108 = case shown="True" w74 {
              tunnel: w73 -> [_ w81]
              frame False {
              }
              frame True {
                n109 = call "BusB Raw Data.vi"("BusB Raw Data"=w81) -> ()  [unwired: 10 in, 1 out]
              }
            }
            n110 = Bundle By Name(cluster=w78, "BusB Serial Port"=w75) -> (w77:T28)
          }
          event User Event {
            n111 = event-data() -> ("BusB Visa Resource"=w85:refnum<visa-resource-name>, "BusB Baud Rate"=w86:string)  [unwired: 1 in]
            n112 = Bundle By Name(cluster=w84, "BusB Serial Port"=w85, "BusB Baud Rate"=w86) -> (w83:T28)
          }
          event User Event {
            n113 = event-data() -> ()  [unwired: 1 in, 2 out]
          }
          event User Event {
            n114 = event-data() -> ("BusB Visa Resource in"=w91:refnum<visa-resource-name>)  [unwired: 1 in]
            n115 = call "Acquisition Started.vi"("BusB Visa Resource"=w91) -> ()  [unwired: 10 in, 1 out]
            n116 = call "Status Updated.vi"("Status"="Acquiring...") -> ()  [unwired: 10 in, 1 out]
          }
          event User Event {
            w97 = -1  # Timeout case will cease execution
            n117 = event-data() -> ()  [unwired: 1 in, 2 out]
            n118 = Unbundle By Name(w96) -> ("BusB Serial Port"=w95:refnum<visa-resource-name>)
            n119 = VISA Close(VISA resource name=w95) -> (error out=w94:errorcluster)  [unwired: 1 in]
          }
        }
        n120 = call-dynamic "Delacor_lib_QMH_Error Handler - Message Handling Loop.vi"("error in"=w63, "Ignore Errors (Runtime)"=w62, "Message Queue in"=w64) -> ()  [unwired: 7 in, 2 out]
      }
      n121 = while {
        tunnel: w37 -> [w98]
        shift-right: [w101] -> w46
        shift-left: w45 -> [w102]
        tunnel: [w103] -> w48
        tunnel: w44 -> [w99]
        stop <- w100 stop-if-true
        # "Event Handling Loop"
        n122 = event "DQMH_EVENT_MAIN" shown="[9] <FINS3-E BusB Data Acquisition and Decoding Request Events.Initialize FINS for FTR>: User Event" {
          selector: w102 -> [_ _ _ _ _ _ _ _ _ _ _]
          dyn-events: [_ _ _ _ _ _ _ _ _ _ _] -> w101
          timeout: _ -> [_ _ _ _ _ _ _ _ _ _ _]
          tunnel: [_ _ _ _ TRUE ("Discard?") _ _ _ _ _ _] -> w100
          tunnel: w98 -> [_ _ _ _ w127 w134 w147 w152 w161 w167 w173]
          tunnel: [_ _ w110 _ w130 w136 w142 w154 w155 w162 w168] -> w104
          tunnel: w99 -> [_ _ _ _ _ w133 _ _ _ _ _]
          event User Event {
            # "Show the panel of this VI, and send a status updated message to let listeners know."
            # "Another Module called the \"Show Panel\" API Method."
            n123 = event-data() -> ()  [unwired: 1 in, 1 out]
            n124 = control-ref of="This VI"() -> (w106:refnum<vi>)
            n125 = call "Open VI Panel.vi"("VI"=w106) -> ()  [unwired: 10 in, 1 out]
            n126 = call "Status Updated.vi"("Status"="Panel shown." ("format string")) -> ()  [unwired: 10 in, 1 out]
          }
          event User Event {
            # "Hide the panel of this VI, and send a status updated message to let listeners know."
            # "Another Module called the \"Hide Panel\" API Method."
            n127 = event-data() -> ()  [unwired: 1 in, 1 out]
            n128 = control-ref of="This VI"() -> (w108:refnum<vi>)
            n129 = call "Hide VI Panel.vi"("VI"=w108) -> ()  [unwired: 10 in, 1 out]
            n130 = call "Status Updated.vi"("Status"="Panel hidden." ("format string")) -> ()  [unwired: 10 in, 1 out]
          }
          event User Event {
            # "Another Module called the \"Get Module Execution Status\" API Method."
            n131 = event-data() -> ()  [unwired: 1 in, 1 out]
            n132 = call "Update Module Execution Status.vi"("Running?"=TRUE) -> ("error out"=w110:errorcluster)  [unwired: 10 in]
          }
          event User Event {
            # "Another Module called the \"Show Diagram\" API Method. This event is used for debugging."
            n133 = event-data() -> ()  [unwired: 1 in, 1 out]
            n134 = disable-structure shown="RUN_TIME_ENGINE==False" {
              frame condition #0 (active) {
                # "functionality not available in exe"
                n135 = invoke class="VI" method="Lock State.Get"() -> (error out=w116:errorcluster, "Get Lock State"=w115:T5, "pwd in cache"=w112:bool)  [unwired: 4 in, 1 out]
                n136 = Equal?(x=T5."Password-protected", y=w115) -> (x = y?=w113:bool)
                n137 = Compound Arithmetic op=AND(w113, invert w112) -> (w111:bool)
                n138 = case shown="False" w111 {
                  tunnel: w116 -> [w119 _]
                  frame False {
                    n139 = property class="VI"(error in=w119, "BDWin.Open"=TRUE ("Block Diagram Window:Open")) -> ()  [unwired: 1 in, 2 out]
                    n140 = call "Status Updated.vi"("Status"="Block Diagram shown." ("format string")) -> ()  [unwired: 10 in, 1 out]
                  }
                  frame True {
                    # "Password-protected VI, and the password is not in the cache. Do not show the diagram."
                  }
                }
              }
              frame condition #1 {
              }
            }
          }
          event User Event {
            # "The Stop Module Event can get fired from the Exit message in the MHL. The queue gets destroyed in that case. If the queue no longer exists, the Enqueue Exit as a priority message will return error 1. It is safe to ignore, because the module is already exiting."
            # "Another Module called the \"Stop Module\" API Method  or the Message Handling Loop below."
            n141 = event-data() -> ("Origin"=w120:string, "Exit via Stop Module Req?"=w123:bool, "Wait for Module to stop?"=w122:bool)  [unwired: 1 in]
            n142 = local write "Status"(w120) -> ()
            n143 = Bundle By Name(cluster=T6 {"Origin"="", "Exit via Stop Module Req?"=FALSE, "Wait for Module to stop?"=FALSE} ("Stop Argument"), "Exit via Stop Module Req?"=w123, "Wait for Module to stop?"=w122) -> (w121:T6)
            n144 = call-poly <vilib>:"Delacor_lib_QMH_Enqueue Message (poly).vi"("Priority Message? (F)"=TRUE, "Message Data"=w121, "Message"="Exit", "Message Queue in"=w127) -> ("error out"=w131:errorcluster)  [unwired: 6 in, 1 out]
            n145 = call <vilib>:"Clear Errors.vi"("error in (no error)"=w131, "specific error code to clear (0: all)"=1) -> ("error out"=w130:errorcluster)  [unwired: 4 in, 1 out]
          }
          event Panel Close? {
            w135 = TRUE  # Discard the event, the MHL is responsible for closing and stopping this VI.
            # "Hide the panel or send the 'Exit' message if the user clicks the 'X' on the module main VI panel."
            n146 = event-data() -> ()  [unwired: 1 in, 1 out]
            n147 = property class="Module Admin"(reference=w133) -> ("Accessors:External Launch"=w132:bool)  [unwired: 1 in, 2 out]
            n148 = case shown="True" w132 {
              tunnel: w134 -> [_ w140]
              tunnel: [_ w141] -> w136
              frame True {
                # "If externally launched, clicking the 'X' hides the panel, but doesn't close it."
                n149 = control-ref of="This VI"() -> (w137:refnum<vi>)
                n150 = call "Hide VI Panel.vi"("VI"=w137) -> ()  [unwired: 10 in, 1 out]
              }
              frame False {
                # "If run as a stand-alone VI, clicking the panel 'X' stops the VI."
                n151 = call-poly <vilib>:"Delacor_lib_QMH_Enqueue Message (poly).vi"("Priority Message? (F)"=TRUE, "Message"="Exit", "Message Queue in"=w140) -> ("error out"=w141:errorcluster)  [unwired: 7 in, 1 out]
              }
            }
            n152 = event-data("Discard?"=w135) -> ()  [unwired: 1 in, 1 out]
          }
          event User Event {
            # "Another Module called the \"Stop Acquiring\" API Method."
            n153 = event-data() -> ("Boolean"=w143:bool)  [unwired: 1 in]
            n154 = Bundle(cluster=T7 {"Boolean"=FALSE} ("Stop Acquiring Argument"), "Boolean"=w143) -> (w144:T7)
            n155 = call-poly <vilib>:"Delacor_lib_QMH_Enqueue Message (poly).vi"("Message Data"=w144, "Message"="Stop Acquiring", "Message Queue in"=w147) -> ("error out"=w142:errorcluster)  [unwired: 7 in, 1 out]
          }
          event User Event {
            n156 = event-data() -> ("Logging Configuration"=w151:T10, "BusB Hardware Configuration"=w149:T32)  [unwired: 1 in]
            n157 = Bundle By Name(cluster=T8 {"Settings"={"Logging Configuration"={"Log File Base Path"=path "", "TDMS File Reference"=refnum, "Log File Full Path"=path "", "Test Rport Full Path"=path "", "Operator Settings"={"Test Operator"="", "Test Time"=timestamp(0 s since 1904-01-01), "Test Location"="", "Unit Under Test"="", "Test Name"="Functionality Test"}, "Functionality Test Report Template Path"=path "", "BusD Logging"=enum."Limited"}, "BusA Hardware Configuration"={"BusA Serial Port"="", "BusA Baud Rate"="", "BusA Bus Update Rate (Hz)"="", "FCC Parameters"={"ADU Altitude"=0.0, "RA Altitude"=0.0}}, "BusB Hardware Configuration"={"BusB Serial Port"="", "BusB Baud Rate"="460800", "BusB Initialization Parameters"={"FCC Alignment Pkt"={"Latitude"=0.0, "Longitude"=0.0, "Altitude"=0.0, "Start Alignment"=FALSE, "Alignment Time"=0, "Start Navigation"=FALSE, "Init Alg Parameters"=FALSE}}}, "BusD Hardware Configuration"={"FINS3-E BusD Serial Port"="COM4", "FINS3-E BusD Baud Rate"="460800", "FINS3-E BusD Bus Update Rate (Hz)"=""}, "FINS3-E IMU Hardware Configuration"={"FINS3-E IMU Serial Port"="COM3", "FINS3-E IMU Baud Rate"="460800", "FINS3-E IMU Bus Update Rate (Hz)"=""}, "FINS3-E Config Hardware Configuration"={"FINS3-E Config Serial Port"="COM3", "FINS3-E Config Baud Rate"="460800"}, "DSMAC Hardware Configuration"={"DSMAC Serial Port"="COM3", "DSMAC Baud Rate"="460800", "DSMAC Bus Update Rate (Hz)"=""}, "TERCOM Hardware Configuration"={"TERCOM Serial Port"="COM3", "TERCOM Baud Rate"="460800", "TERCOM Bus Update Rate (Hz)"=""}, "A/C Bus Hardware Configuration"={"A/C Bus Serial Port"="COM3", "A/C Bus Baud Rate"="460800", "A/C Bus Bus Update Rate (Hz)"="", "Aircraft Type"=enum."Mirage"}, "GPS Hardware Configuration"={"GPS Serial Port"="", "GPS Baud Rate"="115200"}, "Equipment Resources"={"Fluke DMM 8846A\nSerial Port"="", "CPX400 Serial Port"="", "Temp. Chamber"=""}}, "Update Settings_error"={"status"=FALSE, "code"=0, "source"=""}} ("Settings Updated Argument"), "Settings.Logging Configuration"=w151, "Settings.BusB Hardware Configuration"=w149) -> (w148:T8)
            n158 = call-poly <vilib>:"Delacor_lib_QMH_Enqueue Message (poly).vi"("Message Data"=w148, "Message"="Update Settings", "Message Queue in"=w152) -> ("error out"=w154:errorcluster)  [unwired: 7 in, 1 out]
          }
          event User Event {
            # "Another Module called the \"Start Acquiring\" API Method."
            n159 = event-data() -> ("Wait Notifier"=w157:refnum<notifier>, "wait for reply"=w156:bool)  [unwired: 1 in]
            n160 = Bundle(cluster=T22 {"Wait Notifier"=refnum, "wait for reply"=FALSE} ("Start Acquiring Argument"), "Wait Notifier"=w157, "wait for reply"=w156) -> (w158:T22)
            n161 = call-poly <vilib>:"Delacor_lib_QMH_Enqueue Message (poly).vi"("Message Data"=w158, "Message"="Start Acquiring", "Message Queue in"=w161) -> ("error out"=w155:errorcluster)  [unwired: 7 in, 1 out]
          }
          event User Event {
            # "Another Module called the \"Initialize FINS for FTR\" API Method."
            n162 = event-data() -> ("Boolean"=w163:bool)  [unwired: 1 in]
            n163 = Bundle(cluster=T23 {"Boolean"=FALSE} ("Initialize FINS for FTR Argument"), "Boolean"=w163) -> (w164:T23)
            n164 = call-poly <vilib>:"Delacor_lib_QMH_Enqueue Message (poly).vi"("Message Data"=w164, "Message"="Initialize FINS for FTR", "Message Queue in"=w167) -> ("error out"=w162:errorcluster)  [unwired: 7 in, 1 out]
          }
          event User Event {
            # "Another Module called the \"Initialize FINS for Qualification\" API Method."
            n165 = event-data() -> ("Boolean"=w169:bool)  [unwired: 1 in]
            n166 = Bundle(cluster=T24 {"Boolean"=FALSE} ("Initialize FINS for Qualification Argument"), "Boolean"=w169) -> (w170:T24)
            n167 = call-poly <vilib>:"Delacor_lib_QMH_Enqueue Message (poly).vi"("Message Data"=w170, "Message"="Initialize FINS for Qualification", "Message Queue in"=w173) -> ("error out"=w168:errorcluster)  [unwired: 7 in, 1 out]
          }
        }
        n168 = call-dynamic "Delacor_lib_QMH_Error Handler - Event Handling Loop.vi"("error in"=w104, "Message Queue in"=w98) -> ("dup error in"=w103:errorcluster)  [unwired: 8 in, 1 out]
      }
    }
    frame Error {
      # "Synchronize Caller Events.vi will inform Start Module.vi that the module has launched and will let the code calling Start Module.vi register for broadcasts and would permit the caller receive the broadcast that an error occurred at launch time."
      n169 = call-dynamic "Delacor_lib_QMH_Release Message Queue.vi"("error in"=w358, "Message Queue"=w356) -> ("error out"=w357:errorcluster)  [unwired: 9 in]
      n170 = call "Synchronize Caller Events.vi"("Singleton Module Admin in"=w359) -> ("error out"=w364:errorcluster)  [unwired: 9 in, 1 out]
      n171 = call "Module Name--constant.vi"() -> ("Module Name"=w362:string)  [unwired: 11 in]
      n172 = Format Into String(format string="An error occurred during initialization. %s is no longer running.", w362) -> (resulting string=w360:string)  [unwired: 2 in, 1 out]
      n173 = Merge Errors(w357, w364) -> (w365:errorcluster)
      n174 = call "Error Reported.vi"("Additional Information"=w360, "Error"=w365) -> ()  [unwired: 9 in, 1 out]
    }
  }
  n175 = Merge Errors(w32, w34) -> (w31:errorcluster)
  n176 = call "Close Module.vi"("error in (no error)"=w31, "Module Admin in"=w27) -> ("error out"=w10:errorcluster, "External Launch"=w21:bool, "Module Admin out"=w22:refnum<class "Delacor_lib_QMH_Module Admin.lvclass">)  [unwired: 7 in]
  n177 = Unregister For Events(event registration refnum=w26, error in=w10) -> (error out=w30:errorcluster)
  n178 = case "External Launch?" shown="True" w21 {
    tunnel: w30 -> [_ w366]
    frame False {
    }
    frame True {
      n179 = case shown="No Error" w366 {
        frame No Error {
          n180 = invoke class="VI" method="FP.Close"() -> ()  [unwired: 3 in, 3 out]
        }
        frame Error {
          n181 = invoke class="VI" method="FP.Open"("Activate"=TRUE ("Activate?")) -> ()  [unwired: 4 in, 5 out]
        }
      }
    }
  }
  n182 = local write "Module Admin"(w22) -> ()
  n183 = Unregister For Events(event registration refnum=w11, error in=w10) -> (error out=w8:errorcluster)
  n184 = Unregister For Events(event registration refnum=w12, error in=w10) -> (error out=w9:errorcluster)
  n185 = Merge Errors(w9, w8) -> (→"error out":errorcluster)
